vi "sender.vi"() -> ()   [LabVIEW 2010]
uses:
  ClassA/attribute_class_enum.ctl
  ClassA/ClassA.lvclass
panel:
  in  "sendButton":bool
  in  "stopButton":bool
  in  "attribute class to load":T1
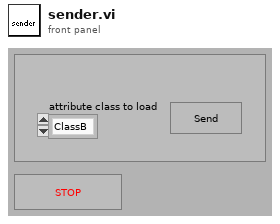
[diagram p1: front panel]
types:
  T1 = typedef "ClassA.lvclass/attribute_class_enum.ctl" = enum16{"ClassB", "ClassC"}
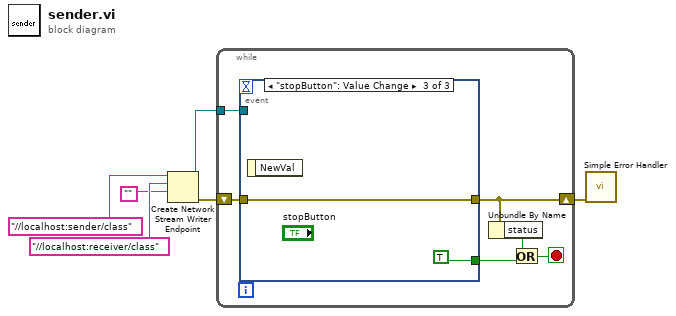
[diagram p0: block diagram]
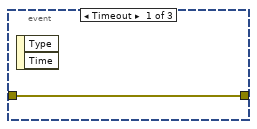
[diagram p2: hidden frame]
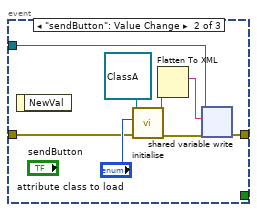
[diagram p3: hidden frame]
diagram:
  n1 = Create Network Stream Writer Endpoint(9:"", 10:"//localhost:receiver/class" ("reader url"), 11:"//localhost:sender/class" ("writer name")) -> (0:w4:errorcluster, 3:w3:refnum<k21>)  [unwired: 3 in]
  n2 = while {
    shift-right: [w10] -> w1
    shift-left: w4 -> [w12]
    tunnel: w3 -> [w11]
    stop <- w8 stop-if-true
    n3 = event shown="[2] \"stopButton\": Value Change" {
      selector: _ -> [_ _ _]
      dyn-events: _ -> [_ _ _]
      timeout: _ -> [_ _ _]
      tunnel: w12 -> [w13 w15 w23]
      tunnel: w11 -> [_ w14 _]
      tunnel: [w13 w16 w23] -> w10
      tunnel: [_ _ TRUE] -> w7
      event Timeout {
        n4 = event-data() -> ()  [unwired: 1 in, 2 out]
      }
      event "sendButton": Value Change {
        n5 = event-data() -> ()  [unwired: 1 in, 1 out]
        n6 = call "initialise.vi"("error in (no error)"=w15, "attribute class to load"="attribute class to load", "ClassA in"=refnum<class "ClassA.lvclass"> refnum ("ClassA.lvclass")) -> ("error out"=w17:errorcluster, "ClassA out"=w20:refnum<class "ClassA.lvclass">)  [unwired: 7 in]
        n7 = Flatten To XML(anything=w20) -> (xml string=w19:string)
        n8 = shared-variable-write(w14, w17, w19) -> (w16:errorcluster)  [unwired: 1 in, 2 out]
      }
      event "stopButton": Value Change {
        n9 = event-data() -> ()  [unwired: 1 in, 1 out]
      }
    }
    n10 = Unbundle By Name(w10) -> ("status"=w9:bool)
    n11 = Or(x=w9, y=w7) -> (x .or. y?=w8:bool)
  }
  n12 = call <vilib>:"Simple Error Handler.vi"("error in (no error)"=w1) -> ()  [unwired: 4 in, 5 out]
